vi "Intan_FilterSettings.vi"(0 "VISA resource name":refnum<visa-resource-name>="COM1", 1 "R_L source":u8(ring) items=["ON-chip", "OFF-chip"], 2 "Lower cutoff":u8(ring)=12 items=["10 Hz", "7.5 Hz", "5.0 Hz", "3.0 Hz", "2.5 Hz", "2.0 Hz", "1.5 Hz", "1.0 Hz", "0.75 Hz", "0.5 Hz", "0.3 Hz", "0.25 Hz", "0.10 Hz"], 3 "Upper cutoff":u8(ring)=10 items=["5.0 kHz", "3.0 kHz", "2.5 kHz", "2.0 kHz", "1.5 kHz", "1.0 kHz", "750 Hz", "500 Hz", "300 Hz", "250 Hz", "200 Hz", "150 Hz", "100 Hz"], 4 "error in":errorcluster) -> (5 "VISA resource name out":refnum<visa-resource-name>, 6 "Text response spi0":string, 7 "error out":errorcluster)   [LabVIEW 2020]
doc: "Use this VI to set Intan RHD2000 series BPF filter parameters. If off-chip R_L is selected, then the lower bandwidth depends on the resistor value connected between aux3 and gnd. For GI applications, we typically use 100 Mohm resistor to set 0.01 Hz low cutoff. If on-chip_R_L is selected, then the low cutoff corresponds to the value chosen in the drop-down menu. \n\nBe sure to call the ADC calibrate command after configuring filters.\n\n(Note that there is currently no option to use off-chip RH_1 and RH_2.)"
panel:
  out "filterSettingsResponse":string
  out "text response spi1":string
  out "return count spi0":u32
  out "return count spi1":u32
  out "ack string":string
  out "string upper":string
  out "string lower":string
  in  "Teensy event char":string="f"
  # "Set BPF cutoffs on RHD2000 chip.\nThis works by sending character 'm' over serial, \nwhich is recognized by Teensy to trigger reading of \ninteger values selected below, then writes the registers 8-13\naccordingly."
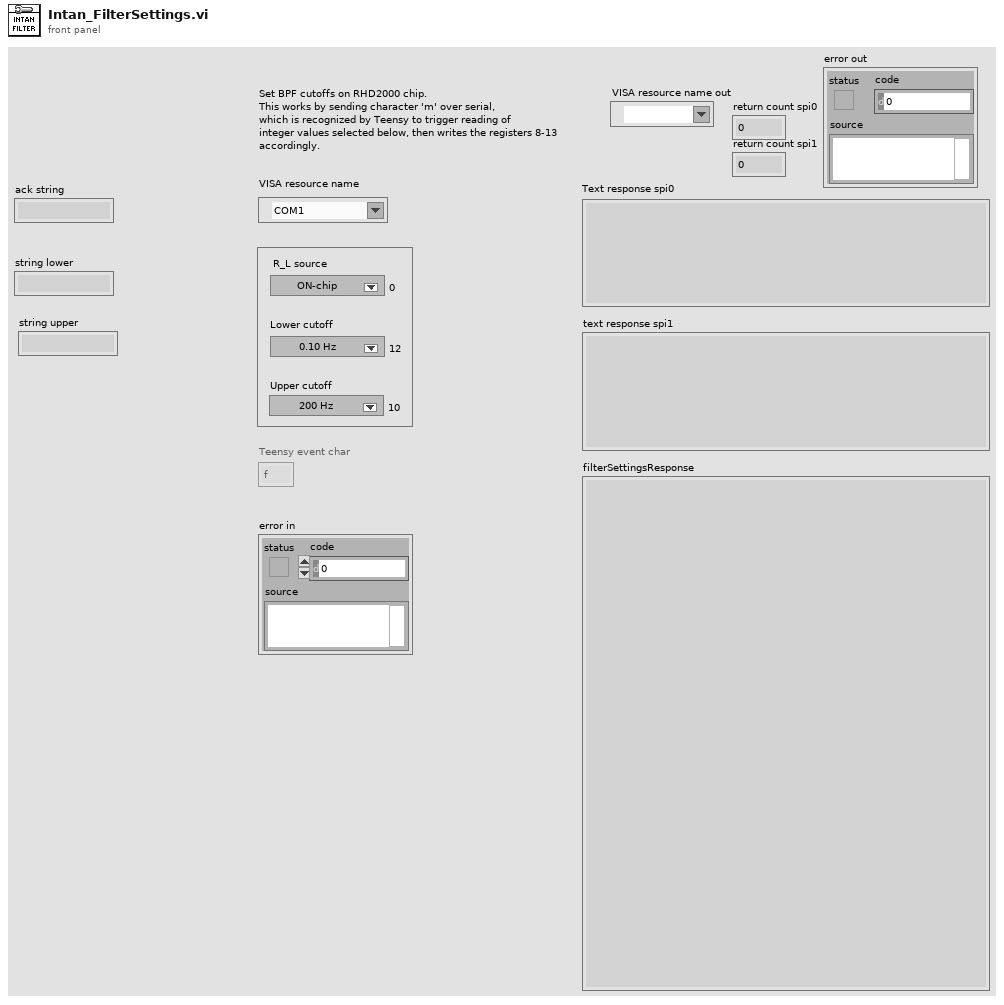
[diagram p1: front panel]
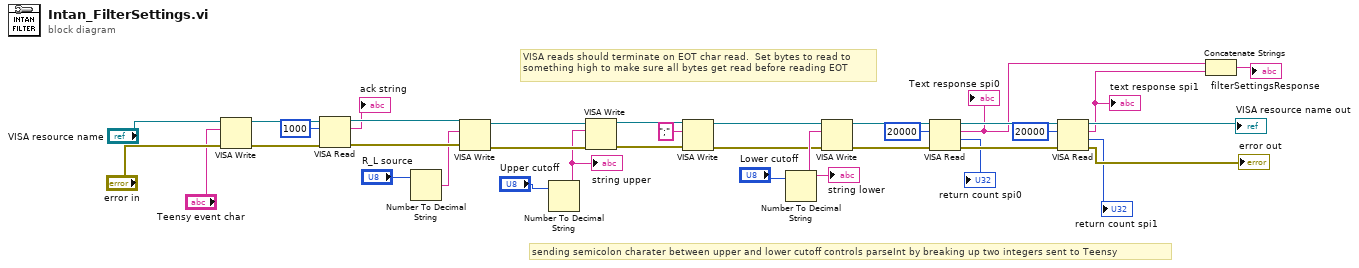
[diagram p0: block diagram]
diagram:
  # "sending semicolon charater between upper and lower cutoff controls parseInt by breaking up two integers sent to Teensy"
  # "VISA reads should terminate on EOT char read.  Set bytes to read to something high to make sure all bytes get read before reading EOT"
  n1 = VISA Write(VISA resource name="VISA resource name", write buffer="Teensy event char", error in (no error)="error in") -> (VISA resource name out=w15:refnum<visa-resource-name>, error out=w14:errorcluster)  [unwired: 1 out]
  n2 = VISA Read(VISA resource name=w15, byte count=u32 1000, error in (no error)=w14) -> (VISA resource name out=w32:refnum<visa-resource-name>, read buffer=→"ack string":string, error out=w31:errorcluster)  [unwired: 1 out]
  n3 = Number To Decimal String(number="R_L source") -> (decimal integer string=w22:string)  [unwired: 1 in]
  n4 = VISA Write(VISA resource name=w32, write buffer=w22, error in (no error)=w31) -> (VISA resource name out=w27:refnum<visa-resource-name>, error out=w28:errorcluster)  [unwired: 1 out]
  n5 = Number To Decimal String(number="Upper cutoff") -> (decimal integer string=w21:string)  [unwired: 1 in]
  "string upper" <- w21
  n6 = VISA Write(VISA resource name=w27, write buffer=w21, error in (no error)=w28) -> (VISA resource name out=w20:refnum<visa-resource-name>, error out=w18:errorcluster)  [unwired: 1 out]
  n7 = VISA Write(VISA resource name=w20, write buffer=";", error in (no error)=w18) -> (VISA resource name out=w19:refnum<visa-resource-name>, error out=w17:errorcluster)  [unwired: 1 out]
  n8 = Number To Decimal String(number="Lower cutoff") -> (decimal integer string=w25:string)  [unwired: 1 in]
  "string lower" <- w25
  n9 = VISA Write(VISA resource name=w19, write buffer=w25, error in (no error)=w17) -> (VISA resource name out=w12:refnum<visa-resource-name>, error out=w11:errorcluster)  [unwired: 1 out]
  n10 = VISA Read(VISA resource name=w12, byte count=u32 20000, error in (no error)=w11) -> (VISA resource name out=w33:refnum<visa-resource-name>, read buffer=w3:string, return count=→"return count spi0":u32, error out=w8:errorcluster)
  "Text response spi0" <- w3
  n11 = VISA Read(VISA resource name=w33, byte count=u32 20000, error in (no error)=w8) -> (VISA resource name out=→"VISA resource name out":refnum<visa-resource-name>, read buffer=w2:string, return count=→"return count spi1":u32, error out=→"error out":errorcluster)
  "text response spi1" <- w2
  n12 = Concatenate Strings(w3, w2) -> (→"filterSettingsResponse":string)
